vi "Enumerate Menus.vi"() -> (3 "Lua menus":T1(c390))   [LabVIEW 2020, in "Lua DevUtil.lvlib"]
uses:
  Lua DevUtil.lvlib
  <vilib>/regexp/Match Regular Expression.xnode
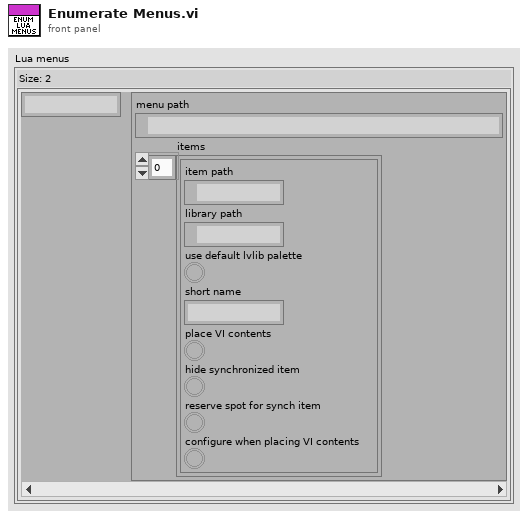
[diagram p1: front panel]
types:
  T1 = map{string, cluster{"menu path":path, "items":cluster{"item path":path, "library path":path, "use default lvlib palette":bool, "short name":string, "place VI contents":bool, "hide synchronized item":bool, "reserve spot for synch item":bool, "configure when placing VI contents":bool}[]}}
  T2 = cluster{"item path":path, "library path":path, "use default lvlib palette":bool, "short name":string, "place VI contents":bool, "hide synchronized item":bool, "reserve spot for synch item":bool, "configure when placing VI contents":bool}[]
  T3 = cluster{"menu path":path, "items":cluster{"item path":path, "library path":path, "use default lvlib palette":bool, "short name":string, "place VI contents":bool, "hide synchronized item":bool, "reserve spot for synch item":bool, "configure when placing VI contents":bool}[]}
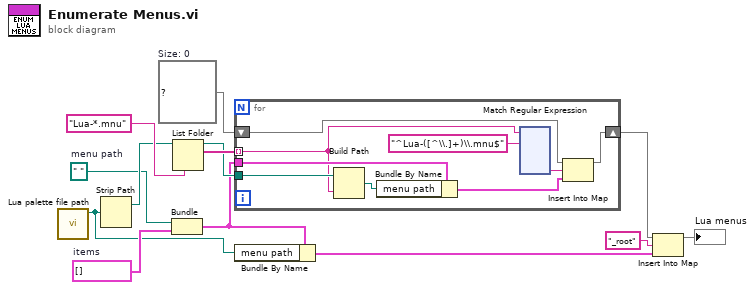
[diagram p0: block diagram]
diagram:
  w7 = T1 {}  # Size: 0
  w9 = path " "  # menu path
  w8 = T2 []  # items
  n1 = call "Lua palette file path.vi"() -> ("palette file path"=w1:path)  [unwired: 11 in]
  n2 = Strip Path(path=w1) -> (stripped path=w11:path)  [unwired: 1 out]
  n3 = Bundle("menu path"=w9, "items"=w8) -> (w3:T3)  [unwired: 1 in]
  n4 = List Folder(path=w11, pattern="Lua-*.mnu") -> (path out=w4:path, filenames=w10:string[])  [unwired: 2 in, 2 out]
  n5 = for {
    shift-right: [w20] -> w6
    shift-left: w7 -> [w18]
    tunnel: w10 -> [w15] mode=indexing
    tunnel: w3 -> [w19]
    tunnel: w4 -> [w16]
    n6 = Build Path(base path=w16, name or relative path=w15) -> (appended path=w14:path)
    n7 = Bundle By Name(cluster=w19, "menu path"=w14) -> (w17:T3)
    n8 = xnode "Match Regular Expression"("input string"=w15, "regular expression"="^Lua-([^\\.]+)\\.mnu$") -> ("submatch 1"=w21:string)  [unwired: 4 in, 5 out]
    n9 = Insert Into Map(map in=w18, key=w21, value=w17) -> (map out=w20:T1)  [unwired: 2 out]
  }
  n10 = Bundle By Name(cluster=w3, "menu path"=w1) -> (w2:T3)
  n11 = Insert Into Map(map in=w6, key="_root", value=w2) -> (map out=→"Lua menus":T1)  [unwired: 2 out]
